vi "Existing_Doc.vi"() -> ()   [LabVIEW 2026]
uses:
  <vilib>/Utility/NIReport.llb/Report Type.ctl
  <vilib>/Utility/NIReport.llb/Append Report Text (str wrap).vi
  <vilib>/Utility/NIReport.llb/NI_report.lvclass
  <vilib>/Utility/NIReport.llb/NI_ReportGenerationCore.lvlib
panel:
  in  "font settings":T1={"Charset (-1)"=-1, "Weight (-1)"=-1, "Name"="", "Size"=" "}
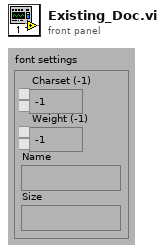
[diagram p1: front panel]
types:
  T1 = cluster{"Charset (-1)":i16, "Weight (-1)":i16, "Name":string, "Size":string}
  T2 = cluster{"position (Excel)":cluster{"row":i32, "column":i32}, "name (Excel)":string, "bookmark (Word)":string}
  T3 = typedef "NI_ReportGenerationCore.lvlib/Report Type.ctl" = enum16{"HTML", "Word", "Excel"}
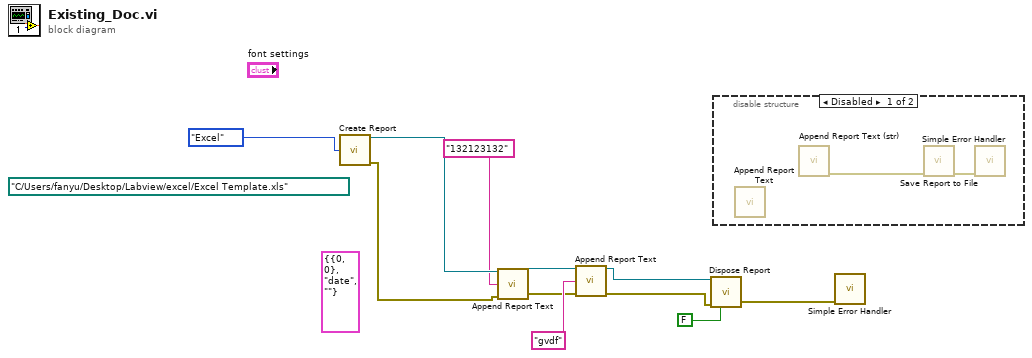
[diagram p0: block diagram]
diagram:
  (unwired) T2 {"position (Excel)"={"row"=0, "column"=0}, "name (Excel)"="date", "bookmark (Word)"=""} ("MS Office parameters")
  (unwired) path "C:/Users/fanyu/Desktop/Labview/excel/Excel Template.xls" ("template (empty)")
  n1 = call <vilib>:"Create Report.vi"("report type"=Report_Type."Excel") -> ("report out"=w8:refnum<class "NI_report.lvclass">, "error out"=w6:errorcluster)  [unwired: 13 in]
  n2 = call-poly <vilib>:"Append Report Text.vi"("report in"=w8, "text"="132123132", "error in (no error)"=w6) -> ("report out"=w5:refnum<class "NI_report.lvclass">, "error out"=w3:errorcluster)  [unwired: 9 in, 2 out]
  n3 = call-poly <vilib>:"Append Report Text.vi"("report in"=w5, "text"="gvdf", "error in (no error)"=w3) -> ("report out"=w2:refnum<class "NI_report.lvclass">, "error out"=w1:errorcluster)  [unwired: 9 in, 2 out]
  n4 = call-dynamic "Dispose Report.vi"("report in"=w2, "error in (no error)"=w1, "close report? (T)"=FALSE ("Close Report? (T)")) -> ("error out"=w10:errorcluster)  [unwired: 12 in]
  n5 = disable-structure shown="Disabled" {
    frame Disabled {
      n6 = call-poly <vilib>:"Append Report Text.vi"() -> ()  [unwired: 12 in, 4 out]
      n7 = call-dynamic "Append Report Text (str).vi"() -> ("error out"=w14:errorcluster)  [unwired: 12 in, 3 out]
      n8 = call-dynamic "Save Report to File.vi"("error in (no error)"=w14) -> ("report file path"=w12:path, "error out"=w13:errorcluster)  [unwired: 12 in, 1 out]
      n9 = call <vilib>:"Simple Error Handler.vi"("error in (no error)"=w13) -> ()  [unwired: 4 in, 5 out]
    }
    frame Enabled {
    }
  }
  n10 = call <vilib>:"Simple Error Handler.vi"("error in (no error)"=w10) -> ()  [unwired: 4 in, 5 out]
